vi "Uninstall All.vi"(7 "Restart Automatically (T)":bool=TRUE, 8 "error in (no error)":errorcluster, 11 "Session in":refnum<k21>) -> (0 "error out":errorcluster, 3 "Session out":refnum<k21>)   [LabVIEW 2017, in "nisyscfg.lvlib"]
doc: "This VI allows you to uninstall all Real-Time software from a system."
uses:
  <vilib>/nisyscfg/nisyscfg.lvlib
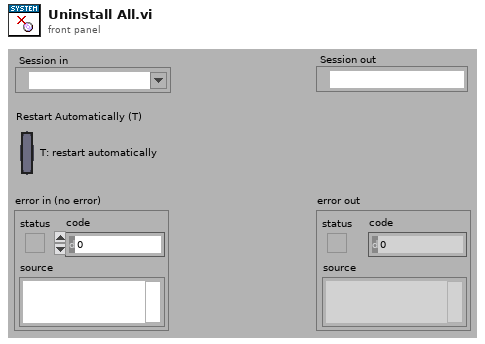
[diagram p1: front panel]
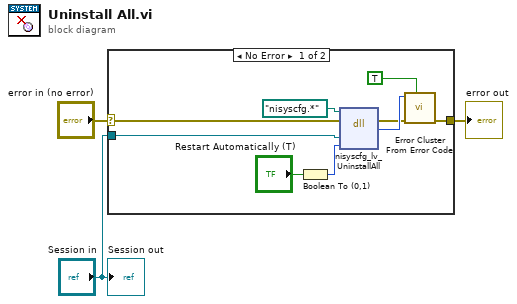
[diagram p0: block diagram]
diagram:
  n1 = case shown="No Error" "error in (no error)" {
    selector: "error in (no error)" -> [w5 w13]
    tunnel: [w4 w13] -> w3
    tunnel: "Session in" -> [w6 _]
    frame No Error {
      n2 = Boolean To (0,1)(Boolean="Restart Automatically (T)") -> (0, 1=w7:i16)
      n3 = dll-call lib="nisyscfg.*" fn="nisyscfg_lv_UninstallAll" label="UninstallAll"(path in=path "nisyscfg.*", error in=w5, "system"=w6, "restartAutomatically"=w7) -> (error out=w11:errorcluster, "result"=w12:i32)  [unwired: 3 in, 1 out]
      n4 = call <vilib>:"Error Cluster From Error Code.vi"("show call chain? (False)"=TRUE, "error in (no error)"=w11, "error code (0)"=w12) -> ("error out"=w4:errorcluster)  [unwired: 6 in]
    }
    frame Error {
    }
  }
  "error out" <- w3
  "Session out" <- "Session in"
